vi "Begin.vi"(11 "Image Size":T1=enum."160x120") -> (0 "error out":errorcluster)   [LabVIEW 2012]
doc: "Called before other user functions, this VI is expected to open initial I/O refnums, load in file data, and do all program initialization. Notice that the <B>error out</B> terminal is simply used for data flow. Wiring it to other structures or subVIs ensures that this VI runs first."
uses:
  <vilib>/Rock Robotics/WPI/Camera/WPI_CameraImageSize.ctl
  <vilib>/Rock Robotics/WPI/DriverStation/WPI_DriverStationRobotMode2.ctl
  <vilib>/Rock Robotics/WPI/Joystick/WPI_JoystickDeviceEnum.ctl
  <vilib>/Rock Robotics/WPI/CAN/Jaguar/SubVIs/WPI_CANJaguar_BrakeCoastMode.ctl
  <vilib>/Rock Robotics/WPI/CAN/Jaguar/SubVIs/WPI_CANJaguar_ControlMode.ctl
  <vilib>/Rock Robotics/WPI/CAN/Jaguar/SubVIs/WPI_CANJaguar_SpeedReference.ctl
  <vilib>/Rock Robotics/WPI/CAN/Jaguar/SubVIs/WPI_CANJaguar_PositionReference.ctl
  <vilib>/Rock Robotics/SystemInterfaces/DIO/FPGA_DIOChannel.ctl
  <vilib>/Rock Robotics/SystemInterfaces/Typedef/FPGA_TypedefDigitalModule.ctl
  <vilib>/Rock Robotics/SystemInterfaces/DIO/FPGA_DIORelayChannel.ctl
  <vilib>/Rock Robotics/SystemInterfaces/Typedef/FPGA_TypedefSolenoidModule.ctl
  <vilib>/Rock Robotics/WPI/Solenoid/WPI_SolenoidChannel.ctl
  Robot Global Data.vi
  <vilib>/Rock Robotics/WPI/MotorControl/WPI_MotorControlOpenCANJaguar.vi
  <vilib>/Rock Robotics/WPI/Solenoid/WPI_SolenoidOpenSingle.vi
  <vilib>/Rock Robotics/WPI/Compressor/WPI_CompressorGetSetRefNum.vi
  <vilib>/Rock Robotics/WPI/Camera/WPI_CameraWhite Balance Values.ctl
  <vilib>/Rock Robotics/WPI/Camera/WPI_CameraExposure Values.ctl
  <vilib>/Rock Robotics/WPI/Camera/WPI_CameraFrameRate.ctl
  <vilib>/Rock Robotics/WPI/RobotDrive/WPI_RobotDriveOpen4MotorWithCANJaguar.vi
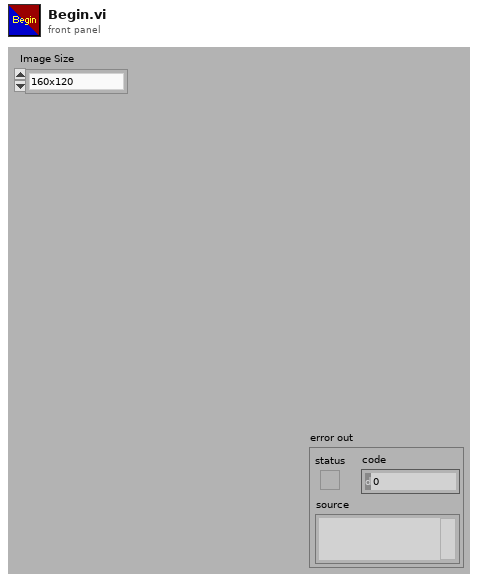
[diagram p1: front panel]
types:
  T1 = typedef "WPI_CameraImageSize.ctl" = enum16{"640x480", "320x240", "160x120"}
  T2 = typedef "WPI_SolenoidChannel.ctl" = enum8{"Solenoid 1", "Solenoid 2", "Solenoid 3", "Solenoid 4", "Solenoid 5", "Solenoid 6", "Solenoid 7", "Solenoid 8", "Invalid"}
  T3 = typedef "FPGA_TypedefSolenoidModule.ctl" = enum16{"Solenoid Module 1", "Solenoid Module 2"}
  T4 = typedef "FPGA_DIORelayChannel.ctl" = enum8{"Relay 1", "Relay 2", "Relay 3", "Relay 4", "Relay 5", "Relay 6", "Relay 7", "Relay 8", "Invalid"}
  T5 = typedef "FPGA_DIOChannel.ctl" = enum8{"DIO 1", "DIO 2", "DIO 3", "DIO 4", "DIO 5", "DIO 6", "DIO 7", "DIO 8", "DIO 9", "DIO 10", "DIO 11", "DIO 12", "DIO 13", "DIO 14", "Invalid"}
  T6 = typedef "FPGA_TypedefDigitalModule.ctl" = enum16{"Digital Module 1", "Digital Module 2"}
  T7 = typedef "WPI_JoystickDeviceEnum.ctl" = enum16{"USB 1", "USB 2", "USB 3", "USB 4", "Kinect 1", "Kinect 2"}
  T8 = typedef "WPI_CANJaguar_PositionReference.ctl" = u8
  T9 = typedef "WPI_CANJaguar_BrakeCoastMode.ctl" = enum8{"Jumper", "Brake", "Coast"}
  T10 = typedef "WPI_CANJaguar_ControlMode.ctl" = enum8{"Percent VBus", "Current", "Speed", "Position", "Voltage"}
  T11 = typedef "WPI_CANJaguar_SpeedReference.ctl" = u8
  T12 = typedef "WPI_DriverStationRobotMode2.ctl" = enum16{"Autonomous Disabled", "Autonomous Enabled", "Teleop Disabled", "Teleop Enabled", "Timeout", "Finish", "Test Disabled", "Test Enabled"}
  T13 = typedef "WPI_JoystickDevRef.ctl" = cluster{"Device":T7}
  T14 = typedef "WPI_SerialPortRef.ctl" = cluster{"DevStatus":errorcluster, "Serial Port Name":refnum<visa-resource-name>}
  T15 = typedef "WPI_CameraFrameRate.ctl" = u32
  T16 = typedef "WPI_CameraExposure Values.ctl" = enum16{"Auto", "Flicker-free 50 Hz", "Flicker-free 60 Hz", "Hold current"}
  T17 = typedef "WPI_CameraWhite Balance Values.ctl" = enum16{"Auto", "Fixed indoor", "Fixed outdoor 1", "Fixed outdoor 2", "Fixed fluorescent 1", "Fixed fluorescent 2", "Hold current"}
  T18 = typedef "WPI_CameraDevRef.ctl" = cluster{"Camera Address":string, "CameraStatus":errorcluster, "Acquire Image Notifier":refnum<notifier>}
  T19 = typedef "WPI_MotorControlDeviceRef.ctl" = cluster{"DeviceStatus":errorcluster, "Type":enum16{"PWM", "CAN"}, "PWM":cluster{"Digital Module":T6, "PWM Channel":T20, "DeadBand":T21}, "CAN":cluster{"Device Number":u8, "Control Mode":T10, "Semaphore":T22, "Max Vout":dbl}, "Invert":bool, "TransformRef":T23, "InvTransformRef":T23}
  T20 = typedef "FPGA_DIOPWMChannel.ctl" = enum8{"PWM 1", "PWM 2", "PWM 3", "PWM 4", "PWM 5", "PWM 6", "PWM 7", "PWM 8", "PWM 9", "PWM 10", "Invalid"}
  T21 = typedef "WPI_PWMDeadband.ctl" = cluster{"Name":string, "maxPositivePwm":i32, "minPositivePwm":i32, "centerPwm":i32, "maxNegativePwm":i32, "minNegativePwm":i32, "angularRange":u16}
  T22 = typedef "Semaphore RefNum" = refnum<k1>
  T23 = typedef "WPI_PWMTransform_ConPane.ctl" = refnum<vi>
  T24 = typedef "WPI_RobotDriveDevRef.ctl" = cluster{"DevStatus":errorcluster, "Motors[]":T19[], "Square Inputs":bool, "Max Output":dbl, "Isochronous":bool}
  T25 = typedef "WPI_CompressorDevRef.ctl" = cluster{"DevStatus":errorcluster, "DigitalInputDevRef":T26, "RelayDevRef":T27}
  T26 = typedef "WPI_DigitalInputDevRef.ctl" = cluster{"DevStatus":errorcluster, "DIO Channel":T5, "Digital Module":T6}
  T27 = typedef "WPI_RelayDevRef.ctl" = cluster{"DevStatus":errorcluster, "Relay Channel":T4, "Digital Module":T6, "Relay Direction":T28}
  T28 = typedef "WPI_RelayDirection.ctl" = enum16{"Both directions", "Forward only", "Reverse only"}
  T29 = typedef "WPI_SolenoidDevRef.ctl" = cluster{"DevStatus":errorcluster, "Solenoid Module":T3, "Forward Solenoid Channel":T2, "Reverse Solenoid Channel":T2}
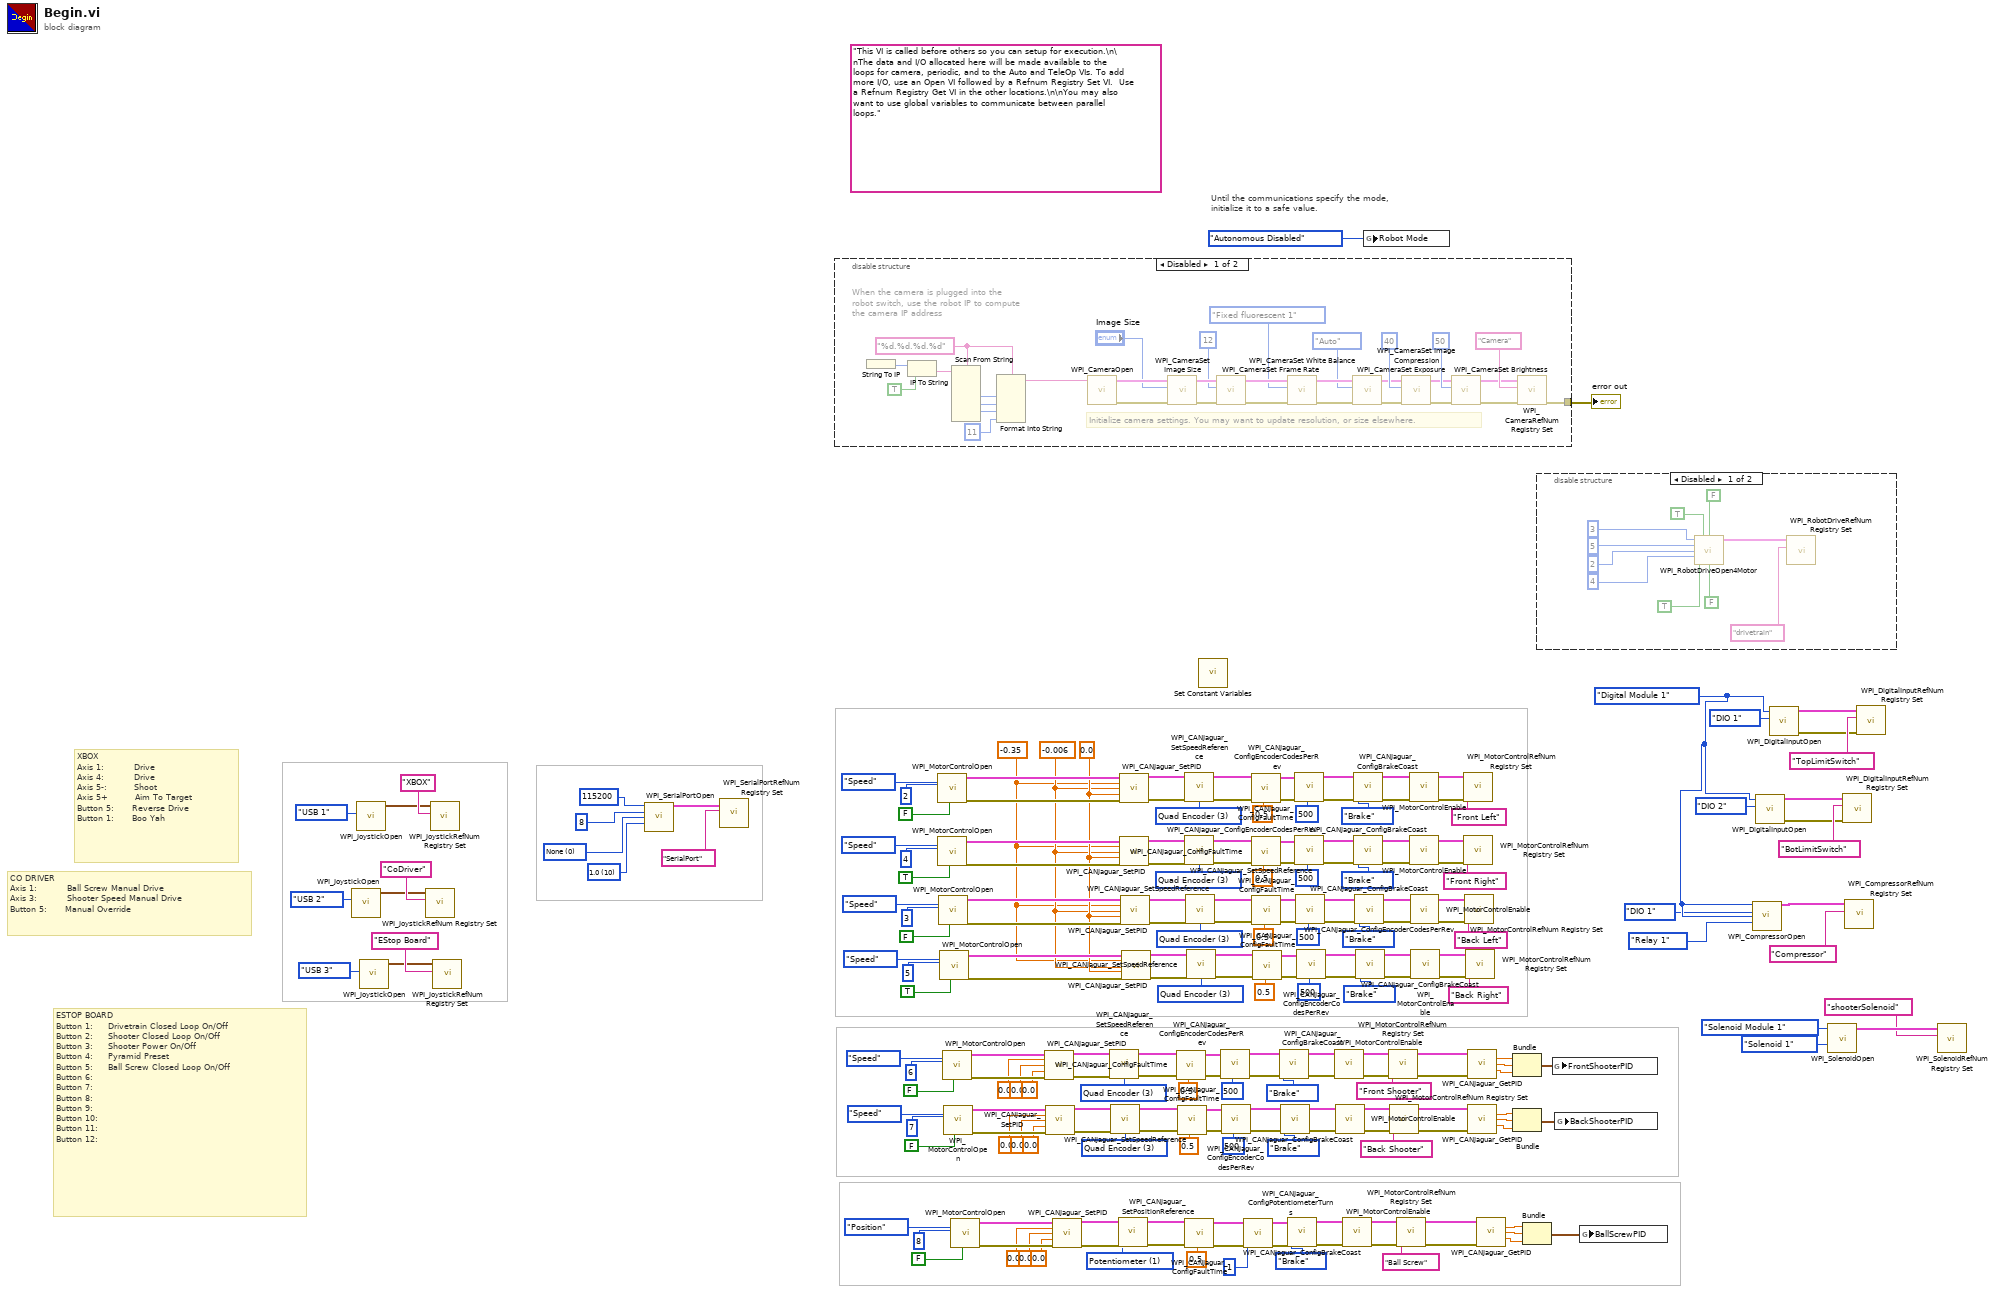
[diagram p0: block diagram]
diagram:
  w8 = FPGA_TypedefDigitalModule."Digital Module 1" ("Digital Module (Module 1)")
  w25 = 0.0 ("D")
  w24 = -0.006 ("I")
  w23 = -0.35 ("P")
  w50 = T8 1 items=["Quad Encoder"=0, "Potentiometer"=1, "None"=255] ("Position Reference")
  w84 = T11 3 items=["Encoder"=0, "Inv Encoder"=2, "Quad Encoder"=3, "None"=255] ("Speed Reference")
  w109 = T11 3 items=["Encoder"=0, "Inv Encoder"=2, "Quad Encoder"=3, "None"=255] ("Speed Reference")
  w131 = T11 3 items=["Encoder"=0, "Inv Encoder"=2, "Quad Encoder"=3, "None"=255] ("Speed Reference")
  w153 = T11 3 items=["Encoder"=0, "Inv Encoder"=2, "Quad Encoder"=3, "None"=255] ("Speed Reference")
  w175 = T11 3 items=["Encoder"=0, "Inv Encoder"=2, "Quad Encoder"=3, "None"=255] ("Speed Reference")
  w197 = T11 3 items=["Encoder"=0, "Inv Encoder"=2, "Quad Encoder"=3, "None"=255] ("Speed Reference")
  w210 = u16 10 items=["1.0"=10, "1.5"=15, "2.0"=20] ("Stop Bits")
  w211 = u16 0 items=["None", "Odd", "Even", "Mark", "Space"] ("Parity")
  (unwired) "This VI is called before others so you can setup for execution.\n\nThe data and I/O allocated here will be made available to the loops for camera, periodic, and to the Auto and TeleOp VIs. To add more I/O, use an Open VI followed by a Refnum Registry Set VI.  Use a Refnum Registry Get VI in the other locations.\n\nYou may also want to use global variables to communicate between parallel loops."
  # "CO DRIVER\nAxis 1:          Ball Screw Manual Drive\nAxis 3:          Shooter Speed Manual Drive\nButton 5:      Manual Override"
  # "XBOX\nAxis 1:          Drive\nAxis 4:          Drive\nAxis 5-:         Shoot\nAxis 5+         Aim To Target\nButton 5:      Reverse Drive\nButton 1:      Boo Yah"
  # "ESTOP BOARD\nButton 1:     Drivetrain Closed Loop On/Off\nButton 2:     Shooter Closed Loop On/Off\nButton 3:     Shooter Power On/Off\nButton 4:     Pyramid Preset\nButton 5:     Ball Screw Closed Loop On/Off\nButton 6:     \nButton 7:\nButton 8:\nButton 9:\nButton 10:\nButton 11:\nButton 12:"
  # "Until the communications specify the mode,\ninitialize it to a safe value."
  n1 = call <vilib>:"WPI_JoystickOpen.vi"("JoystickDevice"=WPI_JoystickDeviceEnum."USB 2") -> ("JoystickDevRef"=w30:T13)  [unwired: 10 in]
  n2 = call <vilib>:"WPI_JoystickOpen.vi"("JoystickDevice"=WPI_JoystickDeviceEnum."USB 1") -> ("JoystickDevRef"=w216:T13)  [unwired: 10 in]
  n3 = call <vilib>:"WPI_JoystickOpen.vi"("JoystickDevice"=WPI_JoystickDeviceEnum."USB 3") -> ("JoystickDevRef"=w27:T13)  [unwired: 10 in]
  n4 = call <vilib>:"WPI_JoystickRefNum Registry Set.vi"("refnum name"="CoDriver", "JoystickDevRef"=w30) -> ()  [unwired: 8 in, 2 out]
  n5 = call <vilib>:"WPI_JoystickRefNum Registry Set.vi"("refnum name"="XBOX", "JoystickDevRef"=w216) -> ()  [unwired: 8 in, 2 out]
  n6 = call <vilib>:"WPI_JoystickRefNum Registry Set.vi"("refnum name"="EStop Board", "JoystickDevRef"=w27) -> ()  [unwired: 8 in, 2 out]
  n7 = call <vilib>:"WPI_SerialPortOpen.vi"("Baud Rate"=u32 115200, "Data Bits"=u16 8, "Parity"=w211, "Stop Bits"=w210) -> ("SerialPortRef"=w209:T14)  [unwired: 10 in, 1 out]
  n8 = call <vilib>:"WPI_SerialPortRefNum Registry Set.vi"("refnum name"="SerialPort", "SerialPortRef"=w209) -> ()  [unwired: 8 in, 2 out]
  n9 = disable-structure shown="Disabled" {
    disable-tunnel: [w219 _] -> w214
    frame Disabled {
      w221 = "%d.%d.%d.%d" ("format string")
      # "When the camera is plugged into the\nrobot switch, use the robot IP to compute\nthe camera IP address"
      # "Initialize camera settings. You may want to update resolution, or size elsewhere."
      n10 = String To IP() -> (0:w228:u32)  [unwired: 1 in]
      n11 = IP To String(1:TRUE ("dot notation? (F)"), 2:w228) -> (0:w226:string)
      n12 = Scan From String(format string=w221, input string=w226) -> (output 1=w225:i32, output 2=w224:i32, output 3=w223:i32)  [unwired: 7 in, 3 out]
      n13 = Format Into String(format string=w221, w225, w224, w223, 11 ("Compression")) -> (resulting string=w220:string)  [unwired: 2 in, 1 out]
      n14 = call <vilib>:"WPI_CameraOpen.vi"("Camera Address"=w220) -> ("error out"=w240:errorcluster, "CameraDevRef"=w241:T18)  [unwired: 1 in, 8 out]
      n15 = call <vilib>:"WPI_CameraSet Image Size.vi"("error in (no error)"=w240, "Image Size"="Image Size", "CameraDevRef"=w241) -> ("error out"=w239:errorcluster, "CameraDevRef Out"=w242:T18)  [unwired: 7 out]
      n16 = call <vilib>:"WPI_CameraSet Frame Rate.vi"("error in (no error)"=w239, "Frame Rate (fps)"=T15 12, "CameraDevRef"=w242) -> ("error out"=w238:errorcluster, "CameraDevRef Out"=w244:T18)  [unwired: 7 out]
      n17 = call <vilib>:"WPI_CameraSet White Balance.vi"("error in (no error)"=w238, "White Balance"=WPI_CameraWhite_Balance_Values."Fixed fluorescent 1", "CameraDevRef"=w244) -> ("error out"=w237:errorcluster, "CameraDevRef Out"=w243:T18)  [unwired: 7 out]
      n18 = call <vilib>:"WPI_CameraSet Exposure.vi"("error in (no error)"=w237, "Exposure"=WPI_CameraExposure_Values."Auto", "CameraDevRef"=w243) -> ("error out"=w236:errorcluster, "CameraDevRef Out"=w246:T18)  [unwired: 7 out]
      n19 = call <vilib>:"WPI_CameraSet Image Compression.vi"("error in (no error)"=w236, "Compression"=40, "CameraDevRef"=w246) -> ("error out"=w235:errorcluster, "CameraDevRef Out"=w245:T18)  [unwired: 7 out]
      n20 = call <vilib>:"WPI_CameraSet Brightness.vi"("error in (no error)"=w235, "Brightness"=50, "CameraDevRef"=w245) -> ("error out"=w233:errorcluster, "CameraDevRef Out"=w234:T18)  [unwired: 7 out]
      n21 = call <vilib>:"WPI_CameraRefNum Registry Set.vi"("error in (no error)"=w233, "refnum name"="Camera", "CameraDevRef"=w234) -> ("error out"=w219:errorcluster)  [unwired: 8 out]
    }
    frame Enabled {
    }
  }
  "error out" <- w214
  n22 = call-poly <vilib>:"WPI_MotorControlOpen.vi"("Invert"=FALSE, "Device Number"=u8 2, "Control Mode"=WPI_CANJaguar_ControlMode."Speed") -> ("error out"=w201:errorcluster, "MotorControlDeviceRef"=w200:T19)  [unwired: 7 in]
  n23 = call-poly <vilib>:"WPI_MotorControlOpen.vi"("Invert"=TRUE, "Device Number"=u8 4, "Control Mode"=WPI_CANJaguar_ControlMode."Speed") -> ("error out"=w179:errorcluster, "MotorControlDeviceRef"=w178:T19)  [unwired: 7 in]
  n24 = call-poly <vilib>:"WPI_MotorControlOpen.vi"("Invert"=FALSE, "Device Number"=u8 3, "Control Mode"=WPI_CANJaguar_ControlMode."Speed") -> ("error out"=w157:errorcluster, "MotorControlDeviceRef"=w156:T19)  [unwired: 7 in]
  n25 = call-poly <vilib>:"WPI_MotorControlOpen.vi"("Invert"=TRUE, "Device Number"=u8 5, "Control Mode"=WPI_CANJaguar_ControlMode."Speed") -> ("error out"=w135:errorcluster, "MotorControlDeviceRef"=w134:T19)  [unwired: 7 in]
  n26 = call-poly <vilib>:"WPI_MotorControlOpen.vi"("Invert"=FALSE, "Device Number"=u8 6, "Control Mode"=WPI_CANJaguar_ControlMode."Speed") -> ("error out"=w113:errorcluster, "MotorControlDeviceRef"=w112:T19)  [unwired: 7 in]
  n27 = call-poly <vilib>:"WPI_MotorControlOpen.vi"("Invert"=FALSE, "Device Number"=u8 7, "Control Mode"=WPI_CANJaguar_ControlMode."Speed") -> ("error out"=w88:errorcluster, "MotorControlDeviceRef"=w87:T19)  [unwired: 7 in]
  n28 = call-poly <vilib>:"WPI_MotorControlOpen.vi"("Invert"=FALSE, "Device Number"=u8 8, "Control Mode"=WPI_CANJaguar_ControlMode."Position") -> ("error out"=w65:errorcluster, "MotorControlDeviceRef"=w64:T19)  [unwired: 7 in]
  n29 = call <vilib>:"WPI_CANJaguar_SetPID.vi"("CAN Jaguar Ref"=w112, "P"=0.0, "I"=0.0, "D"=0.0, "error in (no error)"=w113) -> ("CAN Jaguar Ref Out"=w119:T19, "error out"=w118:errorcluster)  [unwired: 9 in]
  n30 = call <vilib>:"WPI_CANJaguar_SetPID.vi"("CAN Jaguar Ref"=w87, "P"=0.0, "I"=0.0, "D"=0.0, "error in (no error)"=w88) -> ("CAN Jaguar Ref Out"=w94:T19, "error out"=w93:errorcluster)  [unwired: 9 in]
  n31 = call <vilib>:"WPI_CANJaguar_SetPID.vi"("CAN Jaguar Ref"=w64, "P"=0.0, "I"=0.0, "D"=0.0, "error in (no error)"=w65) -> ("CAN Jaguar Ref Out"=w69:T19, "error out"=w68:errorcluster)  [unwired: 9 in]
  n32 = call <vilib>:"WPI_CANJaguar_SetSpeedReference.vi"("error in (no error)"=w118, "Speed Reference"=w109, "CAN Jaguar Ref"=w119) -> ("error out"=w117:errorcluster, "CAN Jaguar Ref Out"=w116:T19)  [unwired: 7 in]
  n33 = call <vilib>:"WPI_CANJaguar_SetSpeedReference.vi"("error in (no error)"=w93, "Speed Reference"=w84, "CAN Jaguar Ref"=w94) -> ("error out"=w92:errorcluster, "CAN Jaguar Ref Out"=w91:T19)  [unwired: 7 in]
  n34 = call <vilib>:"WPI_CANJaguar_SetPositionReference.vi"("error in (no error)"=w68, "Position Reference"=w50, "CAN Jaguar Ref"=w69) -> ("error out"=w67:errorcluster, "CAN Jaguar Ref Out"=w66:T19)  [unwired: 7 in]
  n35 = call <vilib>:"WPI_CANJaguar_SetPID.vi"("CAN Jaguar Ref"=w200, "P"=w23, "I"=w24, "D"=w25, "error in (no error)"=w201) -> ("CAN Jaguar Ref Out"=w207:T19, "error out"=w206:errorcluster)  [unwired: 9 in]
  n36 = call <vilib>:"WPI_CANJaguar_SetPID.vi"("CAN Jaguar Ref"=w178, "P"=w23, "I"=w24, "D"=w25, "error in (no error)"=w179) -> ("CAN Jaguar Ref Out"=w185:T19, "error out"=w184:errorcluster)  [unwired: 9 in]
  n37 = call <vilib>:"WPI_CANJaguar_SetPID.vi"("CAN Jaguar Ref"=w156, "P"=w23, "I"=w24, "D"=w25, "error in (no error)"=w157) -> ("CAN Jaguar Ref Out"=w163:T19, "error out"=w162:errorcluster)  [unwired: 9 in]
  n38 = call <vilib>:"WPI_CANJaguar_SetPID.vi"("CAN Jaguar Ref"=w134, "P"=w23, "I"=w24, "D"=w25, "error in (no error)"=w135) -> ("CAN Jaguar Ref Out"=w141:T19, "error out"=w140:errorcluster)  [unwired: 9 in]
  n39 = call <vilib>:"WPI_CANJaguar_ConfigFaultTime.vi"("error in (no error)"=w117, "Fault Time (s)"=0.5, "CAN Jaguar Ref"=w116) -> ("error out"=w114:errorcluster, "CAN Jaguar Ref Out"=w115:T19)  [unwired: 7 in]
  n40 = call <vilib>:"WPI_CANJaguar_ConfigFaultTime.vi"("error in (no error)"=w92, "Fault Time (s)"=0.5, "CAN Jaguar Ref"=w91) -> ("error out"=w89:errorcluster, "CAN Jaguar Ref Out"=w90:T19)  [unwired: 7 in]
  n41 = call <vilib>:"WPI_CANJaguar_SetSpeedReference.vi"("error in (no error)"=w206, "Speed Reference"=w197, "CAN Jaguar Ref"=w207) -> ("error out"=w205:errorcluster, "CAN Jaguar Ref Out"=w204:T19)  [unwired: 7 in]
  n42 = call <vilib>:"WPI_CANJaguar_SetSpeedReference.vi"("error in (no error)"=w184, "Speed Reference"=w175, "CAN Jaguar Ref"=w185) -> ("error out"=w183:errorcluster, "CAN Jaguar Ref Out"=w182:T19)  [unwired: 7 in]
  n43 = call <vilib>:"WPI_CANJaguar_ConfigFaultTime.vi"("error in (no error)"=w67, "Fault Time (s)"=0.5, "CAN Jaguar Ref"=w66) -> ("error out"=w22:errorcluster, "CAN Jaguar Ref Out"=w21:T19)  [unwired: 7 in]
  n44 = call <vilib>:"WPI_CANJaguar_SetSpeedReference.vi"("error in (no error)"=w162, "Speed Reference"=w153, "CAN Jaguar Ref"=w163) -> ("error out"=w161:errorcluster, "CAN Jaguar Ref Out"=w160:T19)  [unwired: 7 in]
  n45 = call <vilib>:"WPI_CANJaguar_SetSpeedReference.vi"("error in (no error)"=w140, "Speed Reference"=w131, "CAN Jaguar Ref"=w141) -> ("error out"=w139:errorcluster, "CAN Jaguar Ref Out"=w138:T19)  [unwired: 7 in]
  n46 = call "Set Constant Variables.vi"() -> ()  [unwired: 12 in]
  n47 = call <vilib>:"WPI_CANJaguar_ConfigEncoderCodesPerRev.vi"("error in (no error)"=w114, "Encoder Codes Per Rev"=u16 500, "CAN Jaguar Ref"=w115) -> ("error out"=w106:errorcluster, "CAN Jaguar Ref Out"=w105:T19)  [unwired: 7 in]
  n48 = call <vilib>:"WPI_CANJaguar_ConfigEncoderCodesPerRev.vi"("error in (no error)"=w89, "Encoder Codes Per Rev"=u16 500, "CAN Jaguar Ref"=w90) -> ("error out"=w81:errorcluster, "CAN Jaguar Ref Out"=w80:T19)  [unwired: 7 in]
  n49 = call <vilib>:"WPI_CANJaguar_ConfigPotentiometerTurns.vi"("error in (no error)"=w22, "Potentiometer Turns"=u16 1, "CAN Jaguar Ref"=w21) -> ("error out"=w19:errorcluster, "CAN Jaguar Ref Out"=w20:T19)  [unwired: 7 in]
  n50 = call <vilib>:"WPI_CANJaguar_ConfigFaultTime.vi"("error in (no error)"=w205, "Fault Time (s)"=0.5, "CAN Jaguar Ref"=w204) -> ("error out"=w202:errorcluster, "CAN Jaguar Ref Out"=w203:T19)  [unwired: 7 in]
  n51 = call <vilib>:"WPI_CANJaguar_ConfigFaultTime.vi"("error in (no error)"=w183, "Fault Time (s)"=0.5, "CAN Jaguar Ref"=w182) -> ("error out"=w180:errorcluster, "CAN Jaguar Ref Out"=w181:T19)  [unwired: 7 in]
  n52 = call <vilib>:"WPI_CANJaguar_ConfigFaultTime.vi"("error in (no error)"=w161, "Fault Time (s)"=0.5, "CAN Jaguar Ref"=w160) -> ("error out"=w158:errorcluster, "CAN Jaguar Ref Out"=w159:T19)  [unwired: 7 in]
  n53 = call <vilib>:"WPI_CANJaguar_ConfigFaultTime.vi"("error in (no error)"=w139, "Fault Time (s)"=0.5, "CAN Jaguar Ref"=w138) -> ("error out"=w136:errorcluster, "CAN Jaguar Ref Out"=w137:T19)  [unwired: 7 in]
  n54 = call <vilib>:"WPI_CANJaguar_ConfigBrakeCoast.vi"("error in (no error)"=w106, "Brake / Coast Mode"=WPI_CANJaguar_BrakeCoastMode."Brake", "CAN Jaguar Ref"=w105) -> ("error out"=w97:errorcluster, "CAN Jaguar Ref Out"=w98:T19)  [unwired: 7 in]
  n55 = call <vilib>:"WPI_CANJaguar_ConfigBrakeCoast.vi"("error in (no error)"=w81, "Brake / Coast Mode"=WPI_CANJaguar_BrakeCoastMode."Brake", "CAN Jaguar Ref"=w80) -> ("error out"=w72:errorcluster, "CAN Jaguar Ref Out"=w73:T19)  [unwired: 7 in]
  n56 = call <vilib>:"WPI_CANJaguar_ConfigBrakeCoast.vi"("error in (no error)"=w19, "Brake / Coast Mode"=WPI_CANJaguar_BrakeCoastMode."Brake", "CAN Jaguar Ref"=w20) -> ("error out"=w53:errorcluster, "CAN Jaguar Ref Out"=w54:T19)  [unwired: 7 in]
  n57 = call <vilib>:"WPI_CANJaguar_ConfigEncoderCodesPerRev.vi"("error in (no error)"=w202, "Encoder Codes Per Rev"=u16 500, "CAN Jaguar Ref"=w203) -> ("error out"=w194:errorcluster, "CAN Jaguar Ref Out"=w193:T19)  [unwired: 7 in]
  n58 = call <vilib>:"WPI_CANJaguar_ConfigEncoderCodesPerRev.vi"("error in (no error)"=w180, "Encoder Codes Per Rev"=u16 500, "CAN Jaguar Ref"=w181) -> ("error out"=w172:errorcluster, "CAN Jaguar Ref Out"=w171:T19)  [unwired: 7 in]
  n59 = call <vilib>:"WPI_CANJaguar_ConfigEncoderCodesPerRev.vi"("error in (no error)"=w158, "Encoder Codes Per Rev"=u16 500, "CAN Jaguar Ref"=w159) -> ("error out"=w150:errorcluster, "CAN Jaguar Ref Out"=w149:T19)  [unwired: 7 in]
  n60 = call <vilib>:"WPI_CANJaguar_ConfigEncoderCodesPerRev.vi"("error in (no error)"=w136, "Encoder Codes Per Rev"=u16 500, "CAN Jaguar Ref"=w137) -> ("error out"=w128:errorcluster, "CAN Jaguar Ref Out"=w127:T19)  [unwired: 7 in]
  n61 = call <vilib>:"WPI_MotorControlEnable.vi"("error in (no error)"=w97, "CAN Jaguar Ref"=w98) -> ("error out"=w95:errorcluster, "CAN Jaguar Ref Out"=w96:T19)  [unwired: 8 in]
  n62 = call <vilib>:"WPI_MotorControlEnable.vi"("error in (no error)"=w72, "CAN Jaguar Ref"=w73) -> ("error out"=w70:errorcluster, "CAN Jaguar Ref Out"=w71:T19)  [unwired: 8 in]
  n63 = call <vilib>:"WPI_MotorControlEnable.vi"("error in (no error)"=w53, "CAN Jaguar Ref"=w54) -> ("error out"=w51:errorcluster, "CAN Jaguar Ref Out"=w52:T19)  [unwired: 8 in]
  n64 = call <vilib>:"WPI_CANJaguar_ConfigBrakeCoast.vi"("error in (no error)"=w194, "Brake / Coast Mode"=WPI_CANJaguar_BrakeCoastMode."Brake", "CAN Jaguar Ref"=w193) -> ("error out"=w188:errorcluster, "CAN Jaguar Ref Out"=w189:T19)  [unwired: 7 in]
  n65 = call <vilib>:"WPI_CANJaguar_ConfigBrakeCoast.vi"("error in (no error)"=w172, "Brake / Coast Mode"=WPI_CANJaguar_BrakeCoastMode."Brake", "CAN Jaguar Ref"=w171) -> ("error out"=w166:errorcluster, "CAN Jaguar Ref Out"=w167:T19)  [unwired: 7 in]
  n66 = call <vilib>:"WPI_CANJaguar_ConfigBrakeCoast.vi"("error in (no error)"=w150, "Brake / Coast Mode"=WPI_CANJaguar_BrakeCoastMode."Brake", "CAN Jaguar Ref"=w149) -> ("error out"=w144:errorcluster, "CAN Jaguar Ref Out"=w145:T19)  [unwired: 7 in]
  n67 = call <vilib>:"WPI_CANJaguar_ConfigBrakeCoast.vi"("error in (no error)"=w128, "Brake / Coast Mode"=WPI_CANJaguar_BrakeCoastMode."Brake", "CAN Jaguar Ref"=w127) -> ("error out"=w122:errorcluster, "CAN Jaguar Ref Out"=w123:T19)  [unwired: 7 in]
  n68 = global write "Robot Global Data.vi" "Robot Mode"(WPI_DriverStationRobotMode2."Autonomous Disabled" ("Robot Mode")) -> ()
  n69 = call <vilib>:"WPI_MotorControlRefNum Registry Set.vi"("error in (no error)"=w95, "refnum name"="Front Shooter", "MotorControlDevRef"=w96) -> ("error out"=w36:errorcluster, "MotorControlDevRef"=w37:T19)  [unwired: 7 in]
  n70 = call <vilib>:"WPI_MotorControlRefNum Registry Set.vi"("error in (no error)"=w70, "refnum name"="Back Shooter", "MotorControlDevRef"=w71) -> ("error out"=w34:errorcluster, "MotorControlDevRef"=w35:T19)  [unwired: 7 in]
  n71 = call <vilib>:"WPI_MotorControlRefNum Registry Set.vi"("error in (no error)"=w51, "refnum name"="Ball Screw", "MotorControlDevRef"=w52) -> ("error out"=w32:errorcluster, "MotorControlDevRef"=w33:T19)  [unwired: 7 in]
  n72 = call <vilib>:"WPI_MotorControlEnable.vi"("error in (no error)"=w188, "CAN Jaguar Ref"=w189) -> ("error out"=w186:errorcluster, "CAN Jaguar Ref Out"=w187:T19)  [unwired: 8 in]
  n73 = call <vilib>:"WPI_MotorControlEnable.vi"("error in (no error)"=w166, "CAN Jaguar Ref"=w167) -> ("error out"=w164:errorcluster, "CAN Jaguar Ref Out"=w165:T19)  [unwired: 8 in]
  n74 = call <vilib>:"WPI_MotorControlEnable.vi"("error in (no error)"=w144, "CAN Jaguar Ref"=w145) -> ("error out"=w142:errorcluster, "CAN Jaguar Ref Out"=w143:T19)  [unwired: 8 in]
  n75 = call <vilib>:"WPI_MotorControlEnable.vi"("error in (no error)"=w122, "CAN Jaguar Ref"=w123) -> ("error out"=w120:errorcluster, "CAN Jaguar Ref Out"=w121:T19)  [unwired: 8 in]
  n76 = call <vilib>:"WPI_MotorControlRefNum Registry Set.vi"("error in (no error)"=w186, "refnum name"="Front Left", "MotorControlDevRef"=w187) -> ()  [unwired: 7 in, 2 out]
  n77 = call <vilib>:"WPI_MotorControlRefNum Registry Set.vi"("error in (no error)"=w164, "refnum name"="Front Right", "MotorControlDevRef"=w165) -> ()  [unwired: 7 in, 2 out]
  n78 = call <vilib>:"WPI_MotorControlRefNum Registry Set.vi"("error in (no error)"=w142, "refnum name"="Back Left", "MotorControlDevRef"=w143) -> ()  [unwired: 7 in, 2 out]
  n79 = call <vilib>:"WPI_MotorControlRefNum Registry Set.vi"("error in (no error)"=w120, "refnum name"="Back Right", "MotorControlDevRef"=w121) -> ()  [unwired: 7 in, 2 out]
  n80 = call <vilib>:"WPI_CANJaguar_GetPID.vi"("CAN Jaguar Ref"=w37, "error in (no error)"=w36) -> ("P"=w48:dbl, "I"=w46:dbl, "D"=w47:dbl)  [unwired: 9 in, 2 out]
  n81 = call <vilib>:"WPI_CANJaguar_GetPID.vi"("CAN Jaguar Ref"=w35, "error in (no error)"=w34) -> ("P"=w44:dbl, "I"=w42:dbl, "D"=w43:dbl)  [unwired: 9 in, 2 out]
  n82 = call <vilib>:"WPI_CANJaguar_GetPID.vi"("CAN Jaguar Ref"=w33, "error in (no error)"=w32) -> ("P"=w40:dbl, "I"=w38:dbl, "D"=w39:dbl)  [unwired: 9 in, 2 out]
  n83 = Bundle("P"=w48, "I"=w46, "D"=w47) -> (w49:cluster{"P":dbl, "I":dbl, "D":dbl})  [unwired: 1 in]
  n84 = Bundle("P"=w44, "I"=w42, "D"=w43) -> (w45:cluster{"P":dbl, "I":dbl, "D":dbl})  [unwired: 1 in]
  n85 = Bundle("P"=w40, "I"=w38, "D"=w39) -> (w41:cluster{"P":dbl, "I":dbl, "D":dbl})  [unwired: 1 in]
  n86 = disable-structure shown="Disabled" {
    frame Disabled {
      n87 = call-poly <vilib>:"WPI_RobotDriveOpen4Motor.vi"("Rear Left Motor"=u8 3, "Rear Left Motor Inverted"=TRUE, "Rear Right Motor Inverted"=FALSE, "Rear Right Motor"=u8 5 ("Rear Left Motor"), "Front Left Motor"=u8 2 ("Rear Left Motor"), "Front Right Motor"=u8 4 ("Rear Left Motor"), "Front Left Motor Inverted"=TRUE, "Front Right Motor Inverted"=FALSE) -> ("RobotDriveDevRef"=w251:T24)  [unwired: 6 in, 1 out]
      n88 = call <vilib>:"WPI_RobotDriveRefNum Registry Set.vi"("refnum name"="drivetrain", "RobotDriveDevRef"=w251) -> ()  [unwired: 8 in, 2 out]
    }
    frame Enabled {
    }
  }
  n89 = global write "Robot Global Data.vi" "FrontShooterPID"(w49) -> ()
  n90 = global write "Robot Global Data.vi" "BackShooterPID"(w45) -> ()
  n91 = global write "Robot Global Data.vi" "BallScrewPID"(w41) -> ()
  n92 = call <vilib>:"WPI_CompressorOpen.vi"("Pressure Switch Digital Module (Module 1)"=w8, "Pressure Switch DIO Channel"=FPGA_DIOChannel."DIO 1", "Relay Digital Module (Module 1)"=w8, "Relay Channel"=FPGA_DIORelayChannel."Relay 1") -> ("CompressorDevRef"=w9:T25)  [unwired: 10 in, 1 out]
  n93 = call <vilib>:"WPI_DigitalInputOpen.vi"("DIO Channel"=FPGA_DIOChannel."DIO 2", "Digital Module (Module 1)"=w8) -> ("error out"=w11:errorcluster, "DigitalInputDevRef"=w13:T26)  [unwired: 8 in]
  n94 = call <vilib>:"WPI_DigitalInputOpen.vi"("DIO Channel"=FPGA_DIOChannel."DIO 1", "Digital Module (Module 1)"=w8) -> ("error out"=w15:errorcluster, "DigitalInputDevRef"=w17:T26)  [unwired: 8 in]
  n95 = call-poly <vilib>:"WPI_SolenoidOpen.vi"("Solenoid Channel"=WPI_SolenoidChannel."Solenoid 1", "Solenoid Module (Module 1)"=FPGA_TypedefSolenoidModule."Solenoid Module 1") -> ("SolenoidDevRef"=w2:T29)  [unwired: 8 in, 1 out]
  n96 = call <vilib>:"WPI_DigitalInputRefNum Registry Set.vi"("error in (no error)"=w11, "refnum name"="BotLimitSwitch", "DigitalInputDevRef"=w13) -> ()  [unwired: 7 in, 2 out]
  n97 = call <vilib>:"WPI_CompressorRefNum Registry Set.vi"("refnum name"="Compressor", "CompressorDevRef"=w9) -> ()  [unwired: 8 in, 2 out]
  n98 = call <vilib>:"WPI_DigitalInputRefNum Registry Set.vi"("error in (no error)"=w15, "refnum name"="TopLimitSwitch", "DigitalInputDevRef"=w17) -> ()  [unwired: 7 in, 2 out]
  n99 = call <vilib>:"WPI_SolenoidRefNum Registry Set.vi"("refnum name"="shooterSolenoid", "SolenoidDevRef"=w2) -> ()  [unwired: 8 in, 2 out]
